vi "Read Topics.vi"(8 "error in":errorcluster, 11 "System in":refnum<class "System.lvclass">) -> (0 "error out":errorcluster, 2 "Topics":T1[](array[typedef]), 3 "System out":refnum<class "System.lvclass">)   [LabVIEW 2014, in "System.lvclass"]
uses:
  System.lvclass
  Controls/Topic Ref.ctl
  System.lvclass/System.ctl
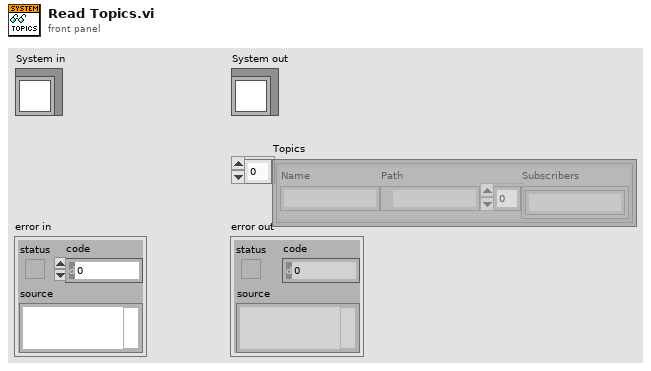
[diagram p1: front panel]
types:
  T1 = typedef "Topic Ref.ctl" = cluster{"Name":string, "Path":path, "Subscribers":string[]}
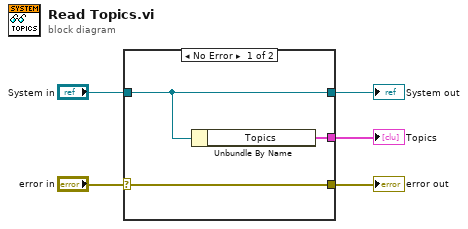
[diagram p0: block diagram]
diagram:
  n1 = case shown="No Error" "error in" {
    selector: "error in" -> [w8 w9]
    tunnel: [w8 w9] -> w4
    tunnel: [w7 w10] -> w2
    tunnel: "System in" -> [w7 w10]
    tunnel: [w6 _] -> w1
    frame No Error {
      n2 = Unbundle By Name(w7) -> ("Topics"=w6:T1[])
    }
    frame Error {
    }
  }
  "error out" <- w4
  "System out" <- w2
  "Topics" <- w1
